vi "Test StringStream Position.vi"() -> ()   [LabVIEW 2020]
uses:
  stream/Stream/Stream.lvclass
  stream/Stream/Stream.lvclass/Stream.ctl
  stream/Stream/Dispatch Sniffer Data.vi
  stream/Stream/Prepared.vi
  stream/Endpoint/Cast Sniffer Callback.vi
  stream/StringStream/StringStream.lvclass
  C:/dev/illuminated-g/lv-stream/stream/Stream/Stream.lvclass
  <vilib>/Utility/error.llb/Error Cluster From Error Code.vi
panel:
  out "Substring":string
  out "error out":errorcluster
  out "Full String":string
  out "Initial Position":i64
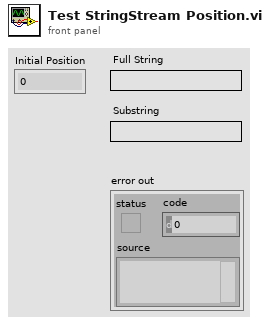
[diagram p1: front panel]
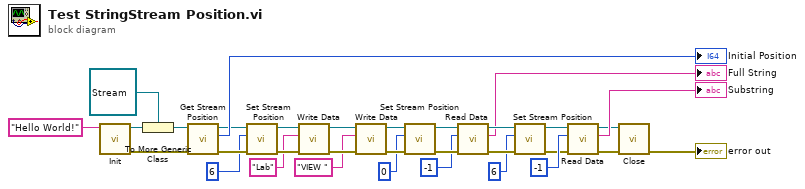
[diagram p0: block diagram]
diagram:
  n1 = call "Init.vi"("Initial String (Empty)"="Hello World!") -> ("error out"=w28:errorcluster, "StringStream out"=w7:refnum<class "StringStream.lvclass">)  [unwired: 9 in]
  n2 = To More Generic Class(target class=refnum<class "Stream.lvclass"> refnum ("Stream in"), reference=w7) -> (generic class reference=w6:refnum<class "Stream.lvclass">)
  n3 = call-dynamic "Get Stream Position.vi"("error in (no error)"=w28, "Stream in"=w6) -> ("error out"=w25:errorcluster, "Position"=→"Initial Position":i64, "Stream out"=w26:refnum<class "Stream.lvclass">)  [unwired: 7 in]
  n4 = call-dynamic "Set Stream Position.vi"("error in (no error)"=w25, "Read Position"=i64 6, "Stream in"=w26) -> ("error out"=w32:errorcluster, "Stream out"=w5:refnum<class "Stream.lvclass">)  [unwired: 7 in]
  n5 = call "Write Data.vi"("error in (no error)"=w32, "Data"="Lab", "Stream in"=w5) -> ("error out"=w31:errorcluster, "Stream out"=w2:refnum<class "Stream.lvclass">)  [unwired: 7 in]
  n6 = call "Write Data.vi"("error in (no error)"=w31, "Data"="VIEW ", "Stream in"=w2) -> ("error out"=w30:errorcluster, "Stream out"=w1:refnum<class "Stream.lvclass">)  [unwired: 7 in]
  n7 = call-dynamic "Set Stream Position.vi"("error in (no error)"=w30, "Read Position"=i64 0, "Stream in"=w1) -> ("error out"=w19:errorcluster, "Stream out"=w20:refnum<class "Stream.lvclass">)  [unwired: 7 in]
  n8 = call "Read Data.vi"("error in (no error)"=w19, "Count"=-1, "Stream in"=w20) -> ("error out"=w16:errorcluster, "Data"=→"Full String":string, "Stream out"=w17:refnum<class "Stream.lvclass">)  [unwired: 6 in]
  n9 = call-dynamic "Set Stream Position.vi"("error in (no error)"=w16, "Read Position"=i64 6, "Stream in"=w17) -> ("error out"=w14:errorcluster, "Stream out"=w13:refnum<class "Stream.lvclass">)  [unwired: 7 in]
  n10 = call "Read Data.vi"("error in (no error)"=w14, "Count"=-1, "Stream in"=w13) -> ("error out"=w10:errorcluster, "Data"=→"Substring":string, "Stream out"=w11:refnum<class "Stream.lvclass">)  [unwired: 6 in]
  n11 = call-dynamic "Close.vi"("error in (no error)"=w10, "Stream in"=w11) -> ("error out"=→"error out":errorcluster)  [unwired: 8 in, 1 out]
